vi "_Raise Launching External Uri Scheme.vi"(4 "WebView2.lvlib:WebView2 Control.lvclass":refnum<class "WebView2 Control.lvclass">, 5 "Event Data":cluster{"sender":refnum<k24>, "e":refnum<k24>}, 6 "Control Ref":refnum<k24>, 7 "Event Common Data":T1) -> ()   [LabVIEW 2025, in "WebView2.lvlib" / "WebView2 Control.lvclass"]
uses:
  WebView2 Control.lvclass
  WebView2 Control.lvclass/WebView2 Control.ctl
  E:/Labview/LV 2023/PPL/PPL Builder/Libs/LV-WebView2/Source/Libs/Microsoft.Web.WebView2.Core.dll
  Libs/Microsoft.Web.WebView2.Core.dll
  Launching External URI Scheme Event Data.ctl
  WebView2 Event Filter Interface/WebView2 Event Filter Interface.lvclass
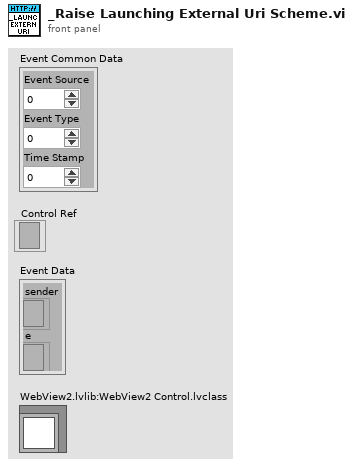
[diagram p1: front panel]
types:
  T1 = cluster{"Event Source":i32, "Event Type":u32, "Time Stamp":u32}
  T2 = typedef "WebView2.lvlib/WebView2 Control.lvclass/Launching External URI Scheme Event Data.ctl" = cluster{"InitiatingOrigin":string, "IsUserInitiated":bool, "Uri":string}
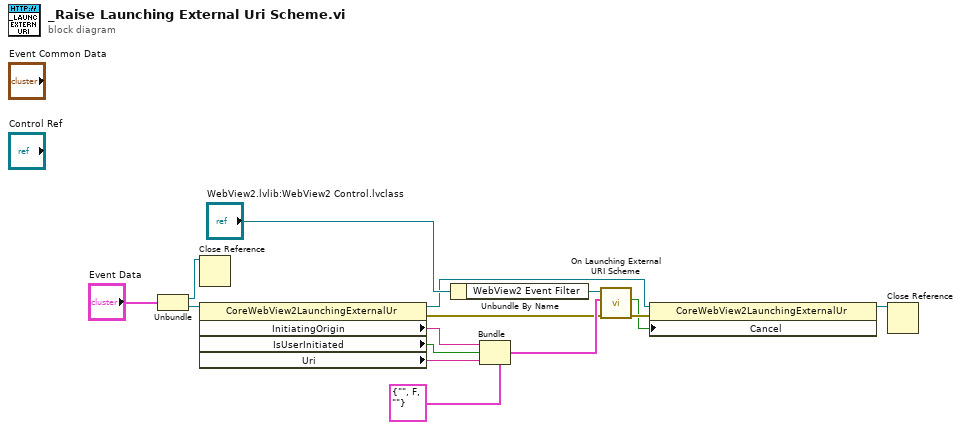
[diagram p0: block diagram]
diagram:
  n1 = Unbundle("Event Data") -> ("sender"=w14:refnum<k24>, "e"=w13:refnum<k24>)
  n2 = Close Reference(reference=w14) -> ()  [unwired: 1 in, 1 out]
  n3 = property class="CoreWebView2LaunchingExternalUr"(reference=w13) -> (reference out=w4:refnum<k24>, error out=w5:errorcluster, "InitiatingOrigin"=w12:string, "IsUserInitiated"=w11:bool, "Uri"=w10:string)  [unwired: 1 in]
  n4 = Unbundle By Name("WebView2.lvlib:WebView2 Control.lvclass") -> ("WebView2 Event Filter"=w7:refnum<class "WebView2 Event Filter Interface.lvclass">)
  n5 = Bundle(cluster=T2 {"InitiatingOrigin"="", "IsUserInitiated"=FALSE, "Uri"=""}, "InitiatingOrigin"=w12, "IsUserInitiated"=w11, "Uri"=w10) -> (w6:T2)
  n6 = call-dynamic "On Launching External URI Scheme.vi"("error in (no error)"=w5, "Data"=w6, "WebView2 Event Filter Interface in"=w7) -> ("error out"=w3:errorcluster, "Cancel"=w2:bool)  [unwired: 7 in]
  n7 = property class="CoreWebView2LaunchingExternalUr"(reference=w4, error in=w3, "Cancel"=w2) -> (reference out=w1:refnum<k24>)  [unwired: 1 out]
  n8 = Close Reference(reference=w1) -> ()  [unwired: 1 in, 1 out]
